vi "setDocumentPath.vi"(8 "error in (no error)":errorcluster, 10 "Document.Path":path, 11 "npoiDocument in":refnum<class "npoiDocument.lvclass">) -> (0 "error out":errorcluster, 3 "npoiDocument out":refnum<class "npoiDocument.lvclass">)   [LabVIEW 2017, in "NPOI_Document.lvlib" / "npoiDocument.lvclass"]
uses:
  npoiDocument.lvclass
  npoiDocument.lvclass/npoiDocument.ctl
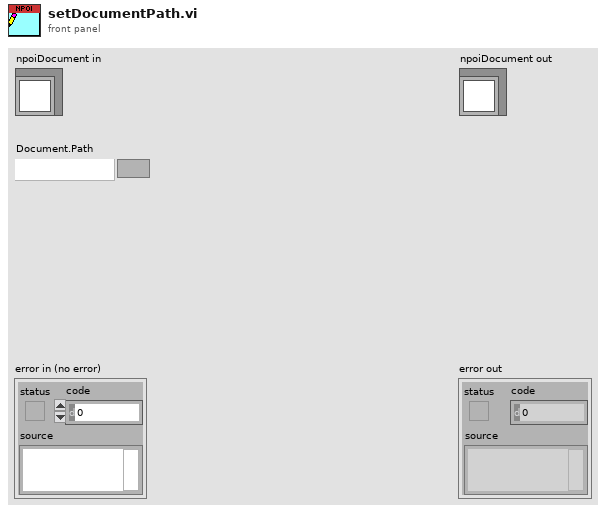
[diagram p1: front panel]
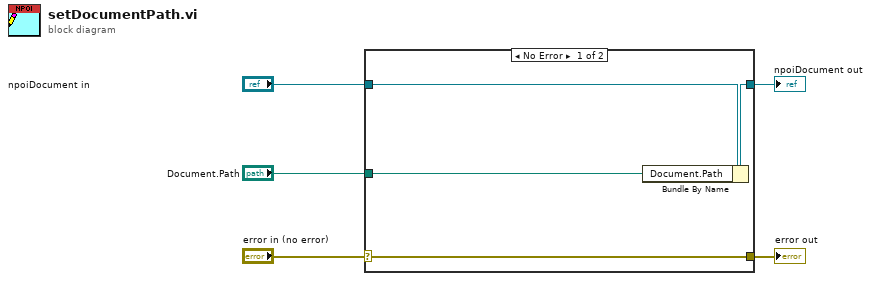
[diagram p0: block diagram]
diagram:
  n1 = case shown="No Error" "error in (no error)" {
    selector: "error in (no error)" -> [w9 w10]
    tunnel: [w9 w10] -> w4
    tunnel: [w7 w11] -> w2
    tunnel: "npoiDocument in" -> [w8 w11]
    tunnel: "Document.Path" -> [w6 _]
    frame No Error {
      n2 = Bundle By Name(cluster=w8, "Document.Path"=w6) -> (w7:refnum<class "npoiDocument.lvclass">)
    }
    frame Error {
    }
  }
  "error out" <- w4
  "npoiDocument out" <- w2
